vi "Zaber Expert - Write Commands and Read Responses.vi"() -> ()   [LabVIEW 2012]
doc: "Another general purpose example. It lets you send one command at a time and displays any responses that come back from the device. This is useful if you want to see responses that aren't caused by requests from the computer, such as manual control or joystick control. This example is similar to the command grid in the Zaber Console.\nThe block diagram is an example of the state machine pattern. It starts in the \"Select Port\" state and waits until you select a port. Then it opens the port in \"Open\" and goes to \"Read\". It stays in \"Read\" and checks for responses until you click a button. \"Write\" sends the command and then goes right back to \"Read\". \"Close\" exits."
uses:
  <instrlib>/ZaberTSeries/Public/Utility/Response.ctl
  Type Definitions/Comandos Zaber.ctl
  <instrlib>/ZaberTSeries/ZaberTSeries.lvlib
panel:
  in  "Comandos":T1 items=["Reset"=0, "Home"=1, "Renumber"=2, "Move Tracking"=8, "Limit Active"=9, "Manual Move Tracking"=10, "Store Current Position"=16, "Return Stored Position"=17, "Move To Stored Position"=18, "Move Absolute"=20, "Move Relative"=21, "Move At Constant Speed"=22, "Stop"=23, "Read Or Write Memory"=35, "Restore Settings"=36, "Set Microstep Resolution"=37, "Set Running Current"=38, "Set Hold Current"=39, "Set Device Mode"=40, "Set Target Speed"=42, "Set Acceleration"=43, "Set Maximum Position"=44, "Set current Position"=45, "Set maximum relative Move"=46, "Set Home Offset"=47, "Set Alias Number"=48, "Set Lock State"=49, "Return Device ID"=50, "Return Firmware Version"=51, "Return Power Supply Voltage"=52, "Return Setting"=53, "Return Status"=54, "Echo Data"=55, "Return current Position"=60, "Error"=255]
  in  "Data":i32
  in  "Device Number":u8=1
  out "Responses":T2[](array[typedef]) {"Command" items=["Constant Speed Tracking"=8, "Echo"=55, "Error"=255, "Home"=1, "Limit Active"=9, "Manual Move Tracking"=10, "Move Absolute"=20, "Move at Constant Speed"=22, "Move Relative"=21, "Renumber"=2, "Restore Settings"=36, "Stop"=23]}
  in  "Stop":bool
  in  "Write":bool
  in  "VISA resource name":refnum<visa-resource-name>
  # "Click the run arrow, and select a COM port. Any \nresponses from Zaber devices will be displayed.\nThis is useful if you want to see responses that\naren't caused by requests from the computer, \nsuch as manual control or joystick control. This\nsample is similar to the command grid in the\nZaber Console."
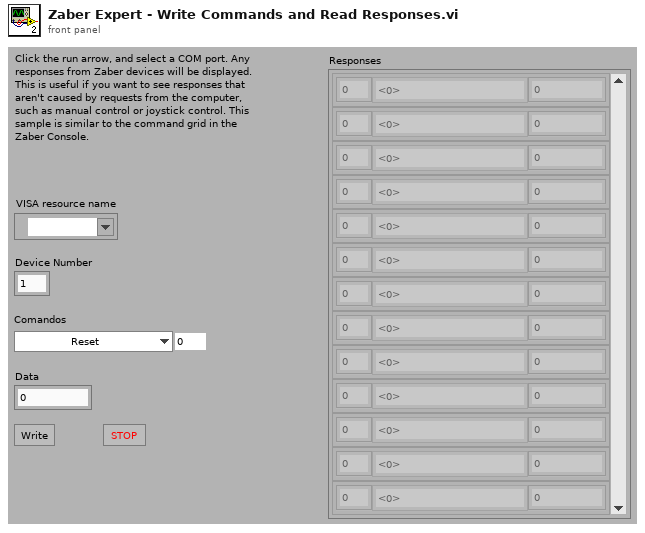
[diagram p1: front panel]
types:
  T1 = typedef "Comandos Zaber.ctl" = u8
  T2 = typedef "ZaberTSeries.lvlib/Response.ctl" = cluster{"Device Number":u8, "Command":u8, "Data":i32}
  T3 = enum8{"Enabled", "Disabled", "Disabled and Grayed Out"}
  T4 = cluster{"Device Number":u8, "Comandos":T1, "Data":i32, "Ignore":i32}
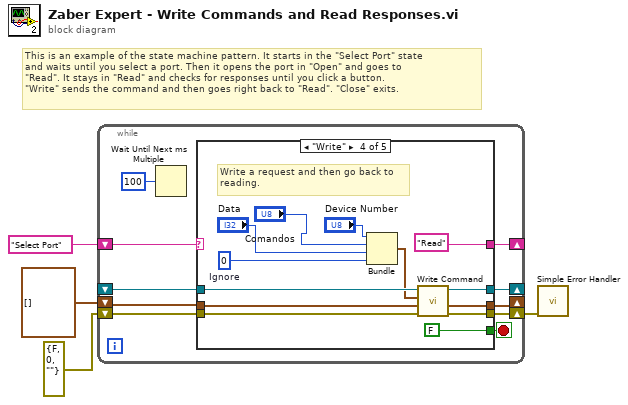
[diagram p0: block diagram]
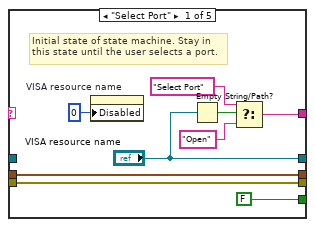
[diagram p2: hidden frame]
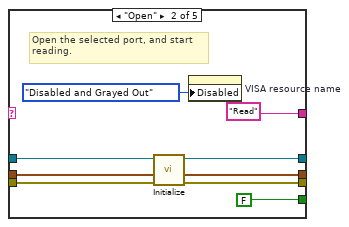
[diagram p3: hidden frame]
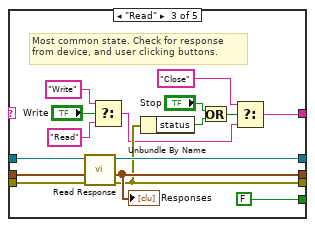
[diagram p4: hidden frame]
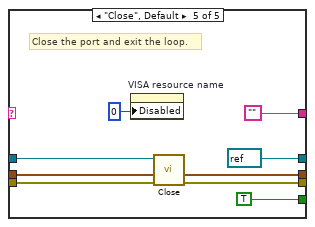
[diagram p5: hidden frame]
diagram:
  # "This is an example of the state machine pattern. It starts in the \"Select Port\" state\nand waits until you select a port. Then it opens the port in \"Open\" and goes to\n\"Read\". It stays in \"Read\" and checks for responses until you click a button.\n\"Write\" sends the command and then goes right back to \"Read\". \"Close\" exits."
  n1 = while {
    shift-right: [w13] -> _
    shift-left: "Select Port" -> [w14]
    shift-right: [w12] -> _
    shift-left: _ -> [w11]
    shift-right: [w10] -> w2
    shift-left: errorcluster {"status"=FALSE, "code"=0, "source"=""} ("error out") -> [w9]
    shift-right: [w7] -> _
    shift-left: T2[] [] ("Responses in") -> [w8]
    stop <- w6 stop-if-true
    n2 = Wait Until Next ms Multiple(millisecond multiple=u32 100) -> ()  [unwired: 1 out]
    n3 = case shown="\"Write\"" w14 {
      tunnel: [w21 "Read" ("f") w33 "Read" ("t") ""] -> w13
      tunnel: ["VISA resource name" w29 w41 w55 refnum<visa-resource-name> refnum ("VISA resource name out")] -> w12
      tunnel: w11 -> [_ w32 w48 w60 w68]
      tunnel: [w17 w31 w38 w56 w66] -> w10
      tunnel: w9 -> [w17 w30 w42 w59 w67]
      tunnel: [w18 w26 w47 w57 w64] -> w7
      tunnel: w8 -> [w18 w25 w46 w58 w65]
      tunnel: [FALSE ("stop") FALSE ("stop") FALSE ("stop") FALSE ("stop") TRUE ("stop")] -> w6
      frame "Select Port" {
        # "Initial state of state machine. Stay in\nthis state until the user selects a port."
        n4 = property on="VISA resource name" class="VISAName"("Disabled"=u8 0) -> ()  [unwired: 2 in, 2 out]
        n5 = Empty String/Path?(string/path="VISA resource name") -> (empty?=w23:bool)
        n6 = Select(t="Select Port", s=w23, f="Open") -> (s? t:f=w21:string)
      }
      frame "Open" {
        # "Open the selected port, and start \nreading."
        n7 = call <instrlib>:"Initialize.vi"("error in (no error)"=w30, "Responses in"=w25, "VISA resource name"=w32) -> ("error out"=w31:errorcluster, "Responses out"=w26:T2[], "VISA resource name out"=w29:refnum<visa-resource-name>)  [unwired: 6 in]
        n8 = property on="VISA resource name" class="VISAName"("Disabled"=T3."Disabled and Grayed Out") -> ()  [unwired: 2 in, 2 out]
      }
      frame "Read" {
        # "Most common state. Check for response\nfrom device, and user clicking buttons."
        n9 = call <instrlib>:"Read Response.vi"("error in (no error)"=w42, "Responses in"=w46, "VISA resource name"=w48) -> ("error out"=w38:errorcluster, "Responses out"=w47:T2[], "VISA resource name out"=w41:refnum<visa-resource-name>)  [unwired: 4 in, 2 out]
        "Responses" <- w47
        n10 = Select(t="Write", s="Write", f="Read" ("t")) -> (s? t:f=w34:string)
        n11 = Unbundle By Name(w38) -> ("status"=w37:bool)
        n12 = Or(x="Stop", y=w37) -> (x .or. y?=w35:bool)
        n13 = Select(t="Close", s=w35, f=w34) -> (s? t:f=w33:string)
      }
      frame "Write" {
        w50 = 0  # Ignore
        # "Write a request and then go back to\nreading."
        n14 = Bundle("Device Number"="Device Number", "Comandos"="Comandos", "Data"="Data", "Ignore"=w50) -> (w53:T4)  [unwired: 1 in]
        n15 = call <instrlib>:"Write Command.vi"("error in (no error)"=w59, "Responses in"=w58, "Request"=w53, "VISA resource name"=w60) -> ("error out"=w56:errorcluster, "Responses out"=w57:T2[], "VISA resource name out"=w55:refnum<visa-resource-name>)  [unwired: 5 in]
      }
      frame "Close", Default {
        # "Close the port and exit the loop."
        n16 = property on="VISA resource name" class="VISAName"("Disabled"=u8 0) -> ()  [unwired: 2 in, 2 out]
        n17 = call <instrlib>:"Close.vi"("error in (no error)"=w67, "Responses in"=w65, "VISA resource name"=w68) -> ("error out"=w66:errorcluster, "Responses out"=w64:T2[])  [unwired: 7 in]
      }
    }
  }
  n18 = call <vilib>:"Simple Error Handler.vi"("error in (no error)"=w2) -> ()  [unwired: 4 in, 5 out]
